vi "Config_Image_Read_ShapeDetect.vi"(8 "error in (no error)":errorcluster) -> (0 "error out":errorcluster)   [LabVIEW 2020]
uses:
  <vilib>/vision/Pattern Matching.llb/IMAQ Match Range Setting.ctl
  <vilib>/Utility/config.llb/Read Key (String).vi
  <vilib>/Utility/config.llb/NI_LVConfig.lvlib
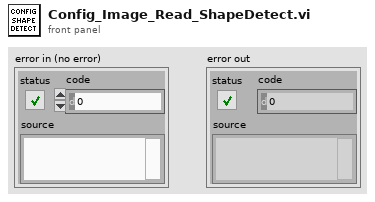
[diagram p1: front panel]
types:
  T1 = typedef "IMAQ Match Range Setting.ctl" = cluster{"Match Constraints":u32, "Min":dbl, "Max":dbl}
  T2 = typedef "Image_Cluster.ctl" = cluster{"Detector_info":cluster{"No. of detectors":dbl, "Detector_Array":string[][], "Detector_Array_Numeric":dbl[][]}, "Corner_info":cluster{"Corner_Array":dbl[][]}, "ROI":cluster{"Corners":cluster{"Global Rectangle":i32[], "Contours":cluster{"ID":enum32{"External", "Internal"}, "Type":u32, "Coordinates":i32[]}[]}[], "Detectors":cluster{"Global Rectangle":i32[], "Contours":cluster{"ID":enum32{"External", "Internal"}, "Type":u32, "Coordinates":i32[]}[]}[]}, "Shape_Detect":cluster{"Match_score":dbl, "Curve Parameters":T3, "Match Options":T4, "Circle Descriptor":cluster{"Min Radius":dbl, "Max Radius":dbl}}, "Path":cluster{"Config":path, "Map":path}, "Map":cluster{"X":i32, "Y":i32}}
  T3 = typedef "IMAQ Curve Parameters.ctl" = cluster{"Extraction Mode":u32, "Edge Threshold":i32, "Edge Filter Size":u32, "Min Length":i32, "Row Search Step Size":i32, "Col Search Step Size":i32, "Max Endpoint Gap":i32, "Closed":bool, "Subpixel":bool}
  T4 = typedef "ShapeDetectionMatchOptions.ctl" = cluster{"Rotation":bool, "Scale":bool, "Occlusion":bool, "Range Settings":T1[]}
  T5 = typedef "NI_LVConfig.lvlib/Config Data RefNum.ctl" = refnum<k1>
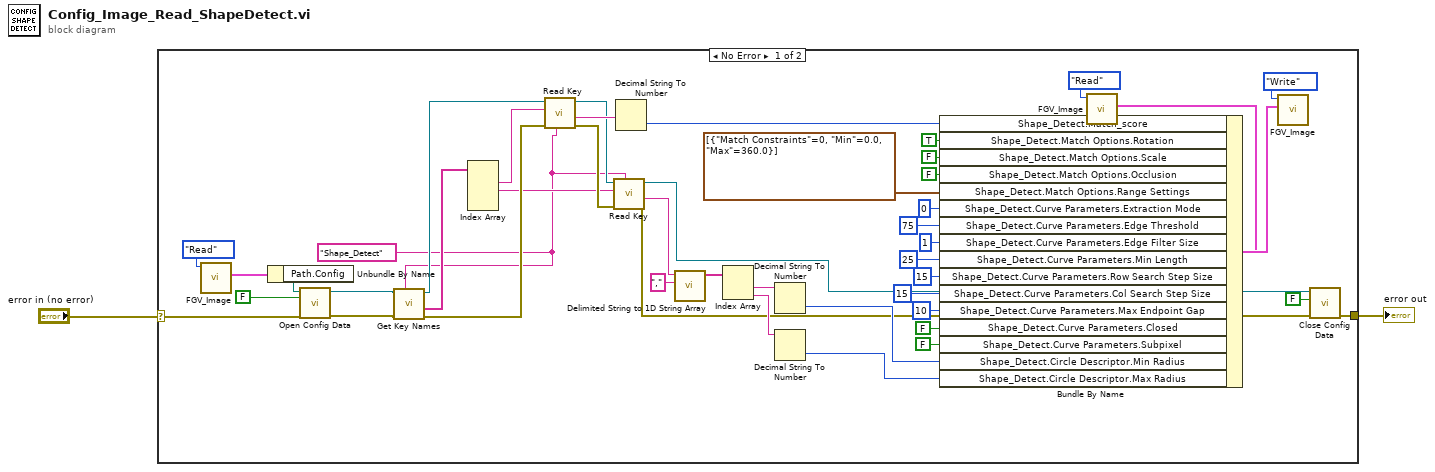
[diagram p0: block diagram]
diagram:
  n1 = case shown="No Error" "error in (no error)" {
    selector: "error in (no error)" -> [w37 w48]
    tunnel: [w47 w48] -> w2
    frame No Error {
      w25 = "Shape_Detect"
      n2 = call "FGV_Image.vi"("Action"=enum16{"Read", "Write", ""}."Read") -> ("Image_Cluster_out"=w45:T2)  [unwired: 10 in]
      n3 = Unbundle By Name(w45) -> ("Path.Config"=w46:path)
      n4 = call <vilib>:"Open Config Data.vi"("error in (no error)"=w37, "create file if necessary (T)"=FALSE, "configuration file path"=w46) -> ("error out"=w36:errorcluster, "refnum"=w35:T5)  [unwired: 6 in, 1 out]
      n5 = call <vilib>:"Get Key Names.vi"("section"=w25, "error in (no error)"=w36, "refnum"=w35) -> ("error out"=w31:errorcluster, "key names"=w34:string[], "refnum out"=w32:T5)  [unwired: 5 in, 1 out]
      n6 = Index Array(array=w34) -> (element #1=w33:string, element #2=w26:string)  [unwired: 4 in, 2 out]
      n7 = call-poly <vilib>:"Read Key.vi"("section"=w25, "error in (no error)"=w31, "key"=w33, "refnum"=w32) -> ("error out"=w28:errorcluster, "value"=w30:string, "refnum out"=w27:T5)  [unwired: 4 in, 1 out]
      n8 = call-poly <vilib>:"Read Key.vi"("section"=w25, "error in (no error)"=w28, "key"=w26, "refnum"=w27) -> ("error out"=w4:errorcluster, "value"=w11:string, "refnum out"=w3:T5)  [unwired: 4 in, 1 out]
      n9 = Decimal String To Number(string=w30) -> (number=w29:i32)  [unwired: 2 in, 1 out]
      n10 = call <vilib>:"Delimited String to 1D String Array.vi"("delimiter"=",", "delimited string"=w11) -> ("string array"=w9:string[])  [unwired: 9 in]
      n11 = Index Array(array=w9) -> (element #1=w8:string, element #2=w7:string)  [unwired: 2 in]
      n12 = Decimal String To Number(string=w8) -> (number=w6:i32)  [unwired: 2 in, 1 out]
      n13 = Decimal String To Number(string=w7) -> (number=w5:i32)  [unwired: 2 in, 1 out]
      n14 = call "FGV_Image.vi"("Action"=enum16{"Read", "Write", ""}."Read") -> ("Image_Cluster_out"=w41:T2)  [unwired: 10 in]
      n15 = Bundle By Name(cluster=w41, "Shape_Detect.Match_score"=w29, "Shape_Detect.Match Options.Rotation"=TRUE, "Shape_Detect.Match Options.Scale"=FALSE, "Shape_Detect.Match Options.Occlusion"=FALSE, "Shape_Detect.Match Options.Range Settings"=T1[] [{"Match Constraints"=0, "Min"=0.0, "Max"=360.0}], "Shape_Detect.Curve Parameters.Extraction Mode"=u32 0, "Shape_Detect.Curve Parameters.Edge Threshold"=75, "Shape_Detect.Curve Parameters.Edge Filter Size"=u32 1, "Shape_Detect.Curve Parameters.Min Length"=25, "Shape_Detect.Curve Parameters.Row Search Step Size"=15, "Shape_Detect.Curve Parameters.Col Search Step Size"=15, "Shape_Detect.Curve Parameters.Max Endpoint Gap"=10, "Shape_Detect.Curve Parameters.Closed"=FALSE, "Shape_Detect.Curve Parameters.Subpixel"=FALSE, "Shape_Detect.Circle Descriptor.Min Radius"=w6, "Shape_Detect.Circle Descriptor.Max Radius"=w5) -> (w42:T2)
      n16 = call "FGV_Image.vi"("Image_Cluster_in"=w42, "Action"=enum16{"Read", "Write", ""}."Write") -> ()  [unwired: 9 in, 1 out]
      n17 = call <vilib>:"Close Config Data.vi"("error in (no error)"=w4, "write file if changed (T)"=FALSE ("write configuration file? (T)"), "refnum"=w3) -> ("error out"=w47:errorcluster)  [unwired: 8 out]
    }
    frame Error {
    }
  }
  "error out" <- w2
